vi "WaveformChart - Colors.vi"(8 "error in (no error)":errorcluster, 10 "Ctl Refnum":refnum<vi>, 11 "Material-Scheme in":refnum<class "Material-Scheme.lvclass">) -> (0 "error out":errorcluster)   [LabVIEW 2021, in "TSC Material Theme.lvlib" / "Material-Scheme.lvclass"]
doc: "Sets the colors of the waveform chart.\n\nColor Rules:\n- Frame, Plot BG: surfaceContainerLowest (preserve transparency)\n- Plot Border: surfaceContainerHighest (preserve transparency)\n- X&Y Scale text: onSurface\n- X&Y Scale gridlines: surfaceContainerHigh (preserve transparency)\n- Digital Numbers: onSurface for text and surfaceContainerHigh for background\n- Plots recolored according to surfaceContainerLowest blending and ratio checking\n\n<b>Code Developed By:</b> +\nDaniel Coons +\nTechnology Service Corporation +\nwww.tsc.com/atcs"
uses:
  Material-Scheme.lvclass
  Material-Scheme.lvclass/Material-Scheme.ctl
  Material SubVIs/Color to HSL.vi
  Material SubVIs/Color to Luminance.vi
  Material SubVIs/HSL to Color.vi
  Material SubVIs/tsc--RGB to Color.vi
  <vilib>/Utility/colorconv.llb/Color to RGB.vi
  Material SubVIs/Material SubVIs.lvlib
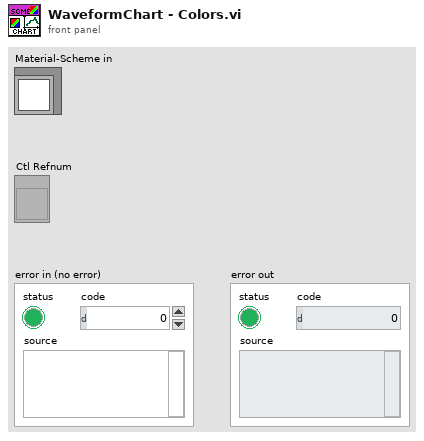
[diagram p1: front panel]
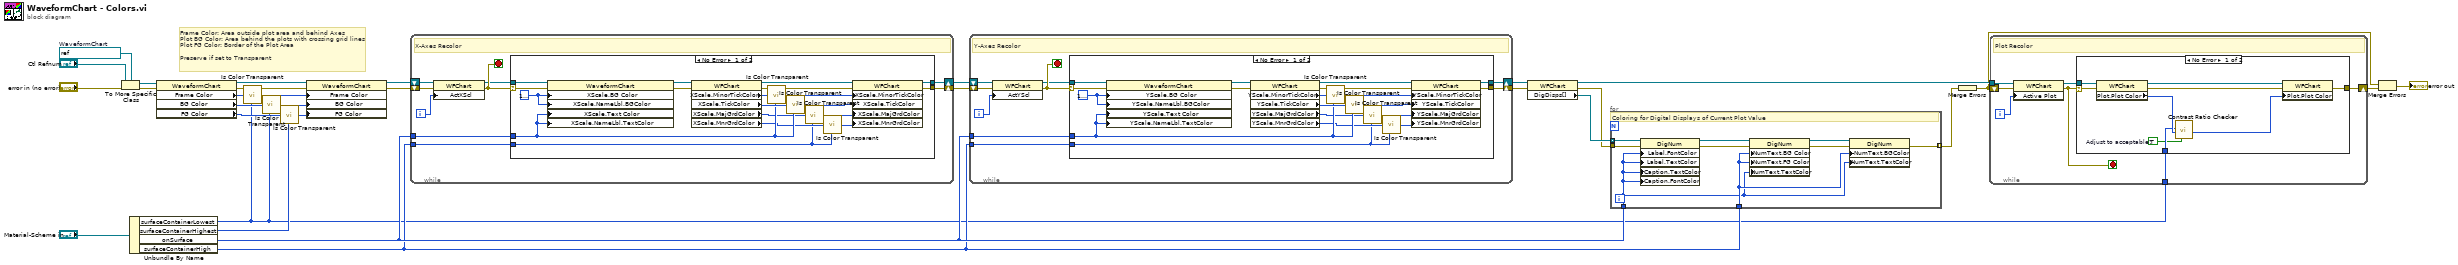
[diagram p0: block diagram]
diagram:
  w29 = refnum<vi> refnum  # WaveformChart
  # "Frame Color: Area outside plot area and behind Axes\nPlot BG Color: Area behind the plots with crossing grid lines\nPlot FG Color: Border of the Plot Area\n\nPreserve if set to Transparent"
  n1 = To More Specific Class(target class=w29, reference="Ctl Refnum", error in="error in (no error)") -> (specific class reference=w30:refnum<vi>, error out=w31:errorcluster)
  n2 = Unbundle By Name("Material-Scheme in") -> ("surfaceContainerLowest"=w1:u32, "surfaceContainerHighest"=w2:u32, "onSurface"=w11:u32, "surfaceContainerHigh"=w10:u32)
  n3 = property class="WaveformChart"(reference=w30, error in=w31) -> (reference out=w16:refnum<vi>, error out=w17:errorcluster, "Frame Color"=w4:u32, "BG Color"=w5:u32, "FG Color"=w6:u32)
  n4 = call "Is Color Transparent.vi"("original color"=w4, "desired color"=w1) -> ("updated color"=w3:u32)  [unwired: 3 in]
  n5 = call "Is Color Transparent.vi"("original color"=w5, "desired color"=w1) -> ("updated color"=w7:u32)  [unwired: 3 in]
  n6 = call "Is Color Transparent.vi"("original color"=w6, "desired color"=w2) -> ("updated color"=w18:u32)  [unwired: 3 in]
  n7 = property class="WaveformChart"(reference=w16, error in=w17, "Frame Color"=w3, "BG Color"=w7, "FG Color"=w18) -> (reference out=w14:refnum<vi>, error out=w15:errorcluster)
  n8 = while {
    shift-right: [w36] -> w13
    shift-left: w15 -> [w40]
    tunnel: w11 -> [w34]
    tunnel: w10 -> [w33]
    shift-right: [w32] -> w12
    shift-left: w14 -> [w39]
    i -> [w38]
    stop <- w37 stop-if-true
    # "X-Axes Recolor"
    n9 = property class="WFChart"(reference=w39, error in=w40, "ActXScl"=w38) -> (reference out=w35:refnum<vi>, error out=w37:errorcluster)
    n10 = case shown="No Error" w37 {
      selector: w37 -> [w59 _]
      tunnel: [w52 _] -> w36
      tunnel: w35 -> [w58 w60]
      tunnel: w34 -> [w48 _]
      tunnel: w33 -> [w42 _]
      tunnel: [w41 w60] -> w32
      frame No Error {
        w57 = u32 16777216 ("X Scale.Name Label.Colors:FG Color")
        n11 = property class="WaveformChart"(reference=w58, error in=w59, "XScale.BG Color"=w57, "XScale.NameLbl.BGColor"=w57, "XScale.Text Color"=w48, "XScale.NameLbl.TextColor"=w48) -> (reference out=w55:refnum<vi>, error out=w56:errorcluster)
        n12 = property class="WFChart"(reference=w55, error in=w56) -> (reference out=w53:refnum<vi>, error out=w54:errorcluster, "XScale.MinorTickColor"=w51:u32, "XScale.TickColor"=w49:u32, "XScale.MajGrdColor"=w46:u32, "XScale.MnrGrdColor"=w45:u32)
        n13 = call "Is Color Transparent.vi"("original color"=w51, "desired color"=w48) -> ("updated color"=w50:u32)  [unwired: 3 in]
        n14 = call "Is Color Transparent.vi"("original color"=w49, "desired color"=w48) -> ("updated color"=w47:u32)  [unwired: 3 in]
        n15 = call "Is Color Transparent.vi"("original color"=w46, "desired color"=w42) -> ("updated color"=w44:u32)  [unwired: 3 in]
        n16 = call "Is Color Transparent.vi"("original color"=w45, "desired color"=w42) -> ("updated color"=w43:u32)  [unwired: 3 in]
        n17 = property class="WFChart"(reference=w53, error in=w54, "XScale.MinorTickColor"=w50, "XScale.TickColor"=w47, "XScale.MajGrdColor"=w44, "XScale.MnrGrdColor"=w43) -> (reference out=w41:refnum<vi>, error out=w52:errorcluster)
      }
      frame Error {
      }
    }
  }
  n18 = while {
    shift-right: [w65] -> w9
    shift-left: w13 -> [w69]
    tunnel: w11 -> [w63]
    tunnel: w10 -> [w62]
    shift-right: [w61] -> w8
    shift-left: w12 -> [w68]
    i -> [w67]
    stop <- w66 stop-if-true
    # "Y-Axes Recolor"
    n19 = property class="WFChart"(reference=w68, error in=w69, "ActYScl"=w67) -> (reference out=w64:refnum<vi>, error out=w66:errorcluster)
    n20 = case shown="No Error" w66 {
      selector: w66 -> [w88 _]
      tunnel: [w81 _] -> w65
      tunnel: w64 -> [w87 w89]
      tunnel: w63 -> [w77 _]
      tunnel: w62 -> [w71 _]
      tunnel: [w70 w89] -> w61
      frame No Error {
        w86 = u32 16777216 ("X Scale.Name Label.Colors:FG Color")
        n21 = property class="WaveformChart"(reference=w87, error in=w88, "YScale.BG Color"=w86, "YScale.NameLbl.BGColor"=w86, "YScale.Text Color"=w77, "YScale.NameLbl.TextColor"=w77) -> (reference out=w84:refnum<vi>, error out=w85:errorcluster)
        n22 = property class="WFChart"(reference=w84, error in=w85) -> (reference out=w82:refnum<vi>, error out=w83:errorcluster, "YScale.MinorTickColor"=w80:u32, "YScale.TickColor"=w78:u32, "YScale.MajGrdColor"=w75:u32, "YScale.MnrGrdColor"=w74:u32)
        n23 = call "Is Color Transparent.vi"("original color"=w80, "desired color"=w77) -> ("updated color"=w79:u32)  [unwired: 3 in]
        n24 = call "Is Color Transparent.vi"("original color"=w78, "desired color"=w77) -> ("updated color"=w76:u32)  [unwired: 3 in]
        n25 = call "Is Color Transparent.vi"("original color"=w75, "desired color"=w71) -> ("updated color"=w73:u32)  [unwired: 3 in]
        n26 = call "Is Color Transparent.vi"("original color"=w74, "desired color"=w71) -> ("updated color"=w72:u32)  [unwired: 3 in]
        n27 = property class="WFChart"(reference=w82, error in=w83, "YScale.MinorTickColor"=w79, "YScale.TickColor"=w76, "YScale.MajGrdColor"=w73, "YScale.MnrGrdColor"=w72) -> (reference out=w70:refnum<vi>, error out=w81:errorcluster)
      }
      frame Error {
      }
    }
  }
  n28 = property class="WFChart"(reference=w8, error in=w9) -> (reference out=w21:refnum<vi>, error out=w23:errorcluster, "DigDisps[]"=w25:refnum<vi>[])
  n29 = for {
    tunnel: w25 -> [w94] mode=indexing
    tunnel: [w93] -> w24 mode=indexing
    tunnel: w11 -> [w90]
    tunnel: w10 -> [w92]
    tunnel: w23 -> [w91]
    # "Coloring for Digital Displays of Current Plot Value"
    n30 = property class="DigNum"(reference=w94, error in=w91, "Label.FontColor"=w90, "Label.TextColor"=w90, "Caption.TextColor"=w90, "Caption.FontColor"=w90) -> (reference out=w97:refnum<vi>, error out=w95:errorcluster)
    n31 = property class="DigNum"(reference=w97, error in=w95, "NumText.BG Color"=w92, "NumText.FG Color"=w92, "NumText.TextColor"=w90) -> (reference out=w98:refnum<vi>, error out=w96:errorcluster)
    n32 = property class="DigNum"(reference=w98, error in=w96, "NumText.BGColor"=w92, "NumText.TextColor"=w90) -> (error out=w93:errorcluster)  [unwired: 1 out]
  }
  n33 = Merge Errors(w24) -> (w19:errorcluster)
  n34 = while {
    tunnel: w21 -> [w104]
    shift-right: [w101] -> w22
    shift-left: w19 -> [w105]
    tunnel: w1 -> [w99]
    i -> [w103]
    stop <- w102 stop-if-true
    # "Plot Recolor"
    n35 = property class="WFChart"(reference=w104, error in=w105, "Active Plot"=w103) -> (reference out=w100:refnum<vi>, error out=w102:errorcluster)
    n36 = case shown="No Error" w102 {
      selector: w102 -> [w114 _]
      tunnel: [w108 _] -> w101
      tunnel: w100 -> [w113 _]
      tunnel: w99 -> [w111 _]
      frame No Error {
        w110 = TRUE  # Adjust to acceptable?
        n37 = property class="WFChart"(reference=w113, error in=w114) -> (reference out=w107:refnum<vi>, error out=w109:errorcluster, "Plot.Plot Color"=w112:u32)
        n38 = call "Contrast Ratio Checker.vi"("Adjust to acceptable?"=w110, "On Color"=w112, "Background Color"=w111) -> ("Adjusted Color"=w106:u32)  [unwired: 6 in, 2 out]
        n39 = property class="WFChart"(reference=w107, error in=w109, "Plot.Plot Color"=w106) -> (error out=w108:errorcluster)  [unwired: 1 out]
      }
      frame Error {
      }
    }
  }
  n40 = Merge Errors(w19, w22) -> (→"error out":errorcluster)
